vi "Get Path Regex.vi"(8 "error in (no error)":errorcluster, 11 "Test Sessions Controller in":refnum<class "Test Sessions Controller.lvclass">) -> (0 "error out":errorcluster, 2 "Path Regex":string, 3 "Test Sessions Controller out":refnum<class "Test Sessions Controller.lvclass">)   [LabVIEW 2020, in "Test Sessions Controller.lvclass"]
uses:
  Test Sessions Controller.lvclass
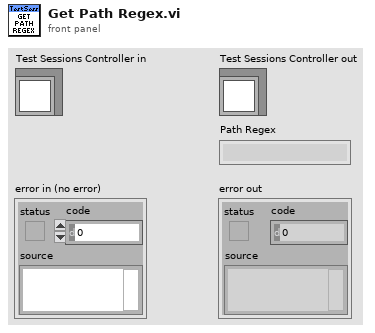
[diagram p1: front panel]
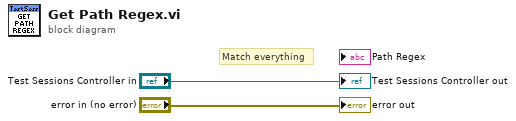
[diagram p0: block diagram]
diagram:
  # "Match everything"
  "error out" <- "error in (no error)"
  "Test Sessions Controller out" <- "Test Sessions Controller in"
